vi "test1.vi"() -> ()   [LabVIEW 2019]
uses:
  <vilib>/measure/NI_MABase.lvlib
panel:
  in  "rate 2":dbl=500.0 format="%#_13g"
  in  "sampling info 6":cluster{"Fs":dbl, "#s":dbl}={"Fs"=2000.0, "#s"=100.0} {"Fs" format="%#_6f"; "#s" format="%#_6f"}
  in  "Back 3":T1={"Channel 1"={" frequency 1"=100, "signal type 1"=enum."Sine Wave", "amplitude 1"=1.5, "offset"=0.0, "phase"=0.0}, "Channel 2"={" frequency 1"=100, "signal type 1"=enum."Sine Wave", "amplitude 1"=1.5, "offset"=0.0, "phase"=90.0}, "Channel 3"={" frequency 1"=100, "signal type 1"=enum."Sine Wave", "amplitude 1"=1.5, "offset"=0, "phase"=180}, "Channel 4"={" frequency 1"=100, "signal type 1"=enum."Sine Wave", "amplitude 1"=1.5, "offset"=0.0, "phase"=270}}
  in  "rate":dbl=50.0 format="%#_13g"
  out "x-y":dbl=2.0449090003967285
  in  "sampling info 5":cluster{"Fs":dbl, "#s":dbl}={"Fs"=500000.0, "#s"=5000.0}
  in  "Back 2":T2={"Channel 1"={" frequency 1"=0, "signal type 1"=enum."Sine Wave", "amplitude 1"=0, "offset"=0.0, "phase"=0.0}, "Channel 2"={" frequency 1"=20000, "signal type 1"=enum."Sine Wave", "amplitude 1"=2.0, "offset"=0.0, "phase"=0.0}, "Channel 3"={" frequency 1"=20000, "signal type 1"=enum."Sine Wave", "amplitude 1"=2.0, "offset"=0, "phase"=0}, "Channel 4"={" frequency 1"=20000, "signal type 1"=enum."Sine Wave", "amplitude 1"=2.0, "offset"=0.0, "phase"=0}}
  in  "stop":bool
  out "Waveform Chart":waveform(dbl)[](graph)=[{"t0"=timestamp(0 s since 1904-01-01), "dt"=0.001, "Y"=[0.0, 1.8369701987210297e-16, -3.6739403974420594e-16, 5.51091059616309e-16, -7.347880794884119e-16, 9.18485099360515e-16, -1.102182119232618e-15, 1.285879139104721e-15, -1.469576158976824e-15, 1.653273178848927e-15, -1.83697019872103e-15, 2.020667218593133e-15, -2.204364238465236e-15, 2.388061258337339e-15, -2.5717582782094417e-15, 2.7554552980815448e-15, -2.9391523179536475e-15, 3.1228493378257506e-15, -3.3065463576978533e-15, 3.4902433775699565e-15, -3.673940397442059e-15, 3.857637417314163e-15, -4.0413344371862654e-15, 4.225031457058369e-15, -4.408728476930472e-15, 4.592425496802575e-15, -4.776122516674678e-15, 4.959819536546781e-15, -5.143516556418884e-15, 5.327213576290988e-15, -5.51091059616309e-15, 5.694607616035194e-15, -5.8783046359072966e-15, 6.0620016557794e-15, -6.245698675651503e-15, 6.429395695523606e-15, -6.613092715395709e-15, 6.7967897352678126e-15, -6.980486755139915e-15, 7.164183775012019e-15, -7.347880794884122e-15, 7.531577814756224e-15, -7.715274834628327e-15, 7.89897185450043e-15, -8.082668874372532e-15, 8.266365894244635e-15, -8.450062914116738e-15, 8.63375993398884e-15, -8.817456953860943e-15, 9.001153973733046e-15, -9.184850993605149e-15, 9.368548013477251e-15, -9.552245033349354e-15, 9.735942053221457e-15, -9.91963907309356e-15, 1.0103336092965662e-14, -1.0287033112837765e-14, 1.0470730132709868e-14, -1.065442715258197e-14, 1.0838124172454073e-14, -1.1021821192326176e-14, 1.1205518212198279e-14, -1.1389215232070381e-14, 1.1572912251942484e-14, -1.1756609271814587e-14, 1.194030629168669e-14, -1.2124003311558792e-14, 1.2307700331430895e-14, -1.2491397351302998e-14, 1.26750943711751e-14, -1.2858791391047203e-14, 1.3042488410919306e-14, -1.3226185430791409e-14, 1.3409882450663511e-14, -1.3593579470535614e-14, 1.3777276490407717e-14, -1.396097351027982e-14, 1.4144670530151922e-14, -1.4328367550024025e-14, 1.4512064569896128e-14, -1.469576158976823e-14, 1.4879458609640333e-14, -1.5063155629512436e-14, 1.524685264938454e-14, -1.543054966925664e-14, 1.5614246689128744e-14, -1.5797943709000847e-14, 1.598164072887295e-14, -1.6165337748745052e-14, 1.6349034768617155e-14, -1.6532731788489258e-14, 1.671642880836136e-14, -1.6900125828233463e-14, 1.7083822848105566e-14, -1.726751986797767e-14, 1.745121688784977e-14, -1.7634913907721874e-14, 1.7818610927593977e-14, -1.800230794746608e-14, 1.8186004967338182e-14]}, {"t0"=timestamp(0 s since 1904-01-01), "dt"=0.001, "Y"=[1.5, -1.5, 1.5, -1.5, 1.5, -1.5, 1.5, -1.5, 1.5, -1.5, 1.5, -1.5, 1.5, -1.5, 1.5, -1.5, 1.5, -1.5, 1.5, -1.5, 1.5, -1.5, 1.5, -1.5, 1.5, -1.5, 1.5, -1.5, 1.5, -1.5, 1.5, -1.5, 1.5, -1.5, 1.5, -1.5, 1.5, -1.5, 1.5, -1.5, 1.5, -1.5, 1.5, -1.5, 1.5, -1.5, 1.5, -1.5, 1.5, -1.5, 1.5, -1.5, 1.5, -1.5, 1.5, -1.5, 1.5, -1.5, 1.5, -1.5, 1.5, -1.5, 1.5, -1.5, 1.5, -1.5, 1.5, -1.5, 1.5, -1.5, 1.5, -1.5, 1.5, -1.5, 1.5, -1.5, 1.5, -1.5, 1.5, -1.5, 1.5, -1.5, 1.5, -1.5, 1.5, -1.5, 1.5, -1.5, 1.5, -1.5, 1.5, -1.5, 1.5, -1.5, 1.5, -1.5, 1.5, -1.5, 1.5, -1.5]}, {"t0"=timestamp(0 s since 1904-01-01), "dt"=0.001, "Y"=[1.8369701987210297e-16, -3.6739403974420594e-16, 5.51091059616309e-16, -7.347880794884119e-16, 9.18485099360515e-16, -1.102182119232618e-15, 1.285879139104721e-15, -1.469576158976824e-15, 1.653273178848927e-15, -1.83697019872103e-15, 2.020667218593133e-15, -2.204364238465236e-15, 2.388061258337339e-15, -2.5717582782094417e-15, 2.7554552980815448e-15, -2.9391523179536475e-15, 3.1228493378257506e-15, -3.3065463576978533e-15, 3.4902433775699565e-15, -3.673940397442059e-15, 3.857637417314163e-15, -4.0413344371862654e-15, 4.225031457058369e-15, -4.408728476930472e-15, 4.592425496802575e-15, -4.776122516674678e-15, 4.959819536546781e-15, -5.143516556418884e-15, 5.327213576290988e-15, -5.51091059616309e-15, 5.694607616035194e-15, -5.8783046359072966e-15, 6.0620016557794e-15, -6.245698675651503e-15, 6.429395695523606e-15, -6.613092715395709e-15, 6.7967897352678126e-15, -6.980486755139915e-15, 7.164183775012019e-15, -7.347880794884122e-15, 7.531577814756224e-15, -7.715274834628327e-15, 7.89897185450043e-15, -8.082668874372532e-15, 8.266365894244635e-15, -8.450062914116738e-15, 8.63375993398884e-15, -8.817456953860943e-15, 9.001153973733046e-15, -9.184850993605149e-15, 9.368548013477251e-15, -9.552245033349354e-15, 9.735942053221457e-15, -9.91963907309356e-15, 1.0103336092965662e-14, -1.0287033112837765e-14, 1.0470730132709868e-14, -1.065442715258197e-14, 1.0838124172454073e-14, -1.1021821192326176e-14, 1.1205518212198279e-14, -1.1389215232070381e-14, 1.1572912251942484e-14, -1.1756609271814587e-14, 1.194030629168669e-14, -1.2124003311558792e-14, 1.2307700331430895e-14, -1.2491397351302998e-14, 1.26750943711751e-14, -1.2858791391047203e-14, 1.3042488410919306e-14, -1.3226185430791409e-14, 1.3409882450663511e-14, -1.3593579470535614e-14, 1.3777276490407717e-14, -1.396097351027982e-14, 1.4144670530151922e-14, -1.4328367550024025e-14, 1.4512064569896128e-14, -1.469576158976823e-14, 1.4879458609640333e-14, -1.5063155629512436e-14, 1.524685264938454e-14, -1.543054966925664e-14, 1.5614246689128744e-14, -1.5797943709000847e-14, 1.598164072887295e-14, -1.6165337748745052e-14, 1.6349034768617155e-14, -1.6532731788489258e-14, 1.671642880836136e-14, -1.6900125828233463e-14, 1.7083822848105566e-14, -1.726751986797767e-14, 1.745121688784977e-14, -1.7634913907721874e-14, 1.7818610927593977e-14, -1.800230794746608e-14, 1.8186004967338182e-14, -1.8369701987210285e-14]}, {"t0"=timestamp(0 s since 1904-01-01), "dt"=0.001, "Y"=[-1.5, 1.5, -1.5, 1.5, -1.5, 1.5, -1.5, 1.5, -1.5, 1.5, -1.5, 1.5, -1.5, 1.5, -1.5, 1.5, -1.5, 1.5, -1.5, 1.5, -1.5, 1.5, -1.5, 1.5, -1.5, 1.5, -1.5, 1.5, -1.5, 1.5, -1.5, 1.5, -1.5, 1.5, -1.5, 1.5, -1.5, 1.5, -1.5, 1.5, -1.5, 1.5, -1.5, 1.5, -1.5, 1.5, -1.5, 1.5, -1.5, 1.5, -1.5, 1.5, -1.5, 1.5, -1.5, 1.5, -1.5, 1.5, -1.5, 1.5, -1.5, 1.5, -1.5, 1.5, -1.5, 1.5, -1.5, 1.5, -1.5, 1.5, -1.5, 1.5, -1.5, 1.5, -1.5, 1.5, -1.5, 1.5, -1.5, 1.5, -1.5, 1.5, -1.5, 1.5, -1.5, 1.5, -1.5, 1.5, -1.5, 1.5, -1.5, 1.5, -1.5, 1.5, -1.5, 1.5, -1.5, 1.5, -1.5, 1.5]}]
  in  "Back":T1={"Channel 1"={" frequency 1"=500, "signal type 1"=enum."Sine Wave", "amplitude 1"=1.5, "offset"=0.0, "phase"=0.0}, "Channel 2"={" frequency 1"=500, "signal type 1"=enum."Sine Wave", "amplitude 1"=1.5, "offset"=0.0, "phase"=90.0}, "Channel 3"={" frequency 1"=500, "signal type 1"=enum."Sine Wave", "amplitude 1"=1.5, "offset"=0, "phase"=180}, "Channel 4"={" frequency 1"=500, "signal type 1"=enum."Sine Wave", "amplitude 1"=1.5, "offset"=0.0, "phase"=270}}
  in  "sampling info 4":cluster{"Fs":dbl, "#s":dbl}={"Fs"=1000.0, "#s"=100.0} {"Fs" format="%#_6f"; "#s" format="%#_6f"}
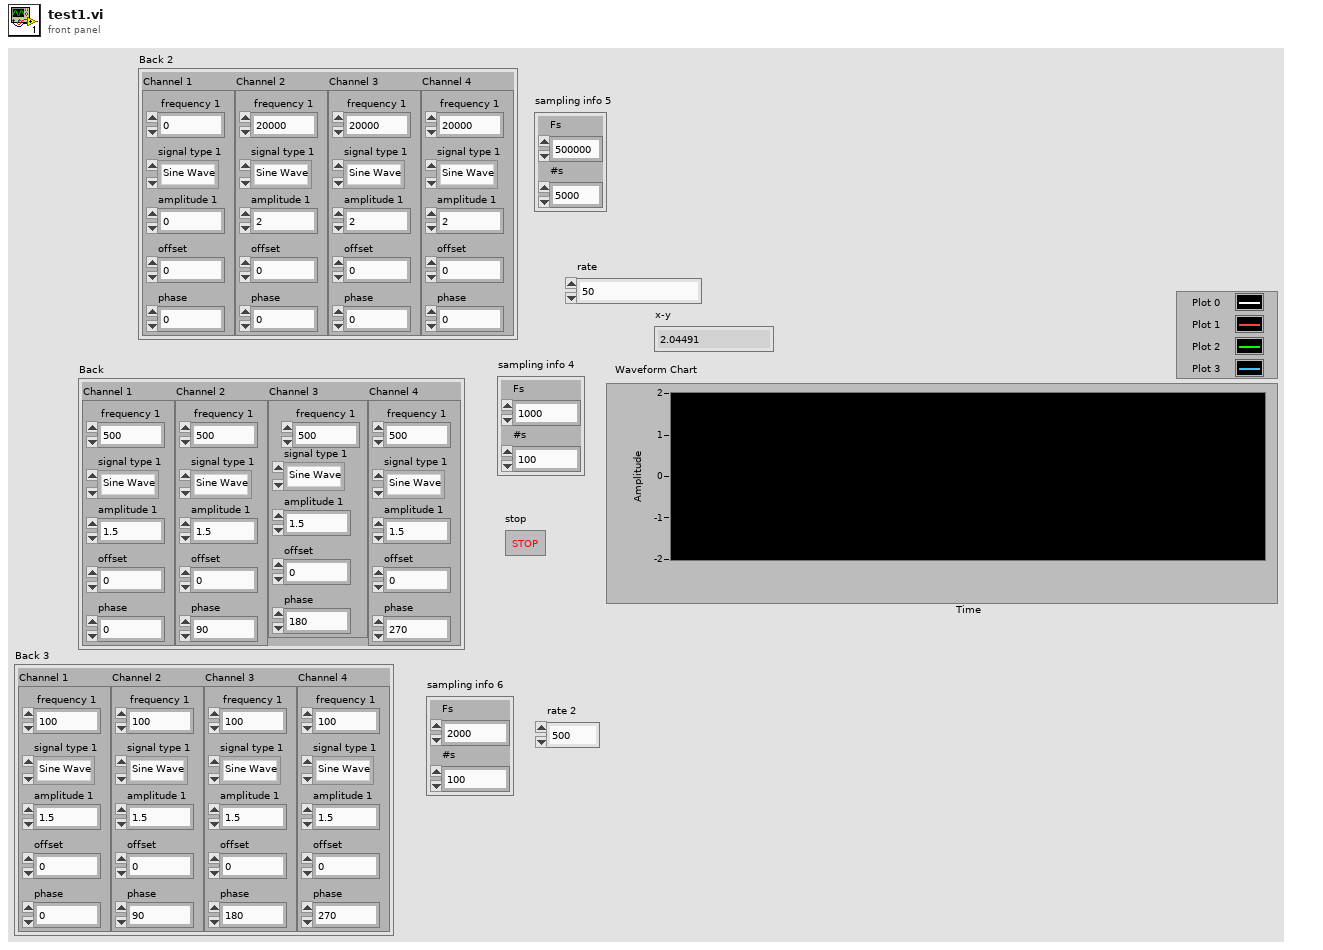
[diagram p1: front panel]
types:
  T1 = cluster{"Channel 1":cluster{" frequency 1":i32, "signal type 1":enum16{"Sine Wave", "Triangle Wave", "Square Wave", "Sawtooth Wave"}, "amplitude 1":dbl, "offset":dbl, "phase":dbl}, "Channel 2":cluster{" frequency 1":i32, "signal type 1":enum16{"Sine Wave", "Triangle Wave", "Square Wave", "Sawtooth Wave"}, "amplitude 1":dbl, "offset":dbl, "phase":dbl}, "Channel 3":cluster{" frequency 1":i32, "signal type 1":enum16{"Sine Wave", "Triangle Wave", "Square Wave", "Sawtooth Wave"}, "amplitude 1":dbl, "offset":i32, "phase":i32}, "Channel 4":cluster{" frequency 1":i32, "signal type 1":enum16{"Sine Wave", "Triangle Wave", "Square Wave", "Sawtooth Wave"}, "amplitude 1":dbl, "offset":dbl, "phase":i32}}
  T2 = cluster{"Channel 1":cluster{" frequency 1":i32, "signal type 1":enum16{"Sine Wave", "Triangle Wave", "Square Wave", "Sawtooth Wave"}, "amplitude 1":i32, "offset":dbl, "phase":dbl}, "Channel 2":cluster{" frequency 1":i32, "signal type 1":enum16{"Sine Wave", "Triangle Wave", "Square Wave", "Sawtooth Wave"}, "amplitude 1":dbl, "offset":dbl, "phase":dbl}, "Channel 3":cluster{" frequency 1":i32, "signal type 1":enum16{"Sine Wave", "Triangle Wave", "Square Wave", "Sawtooth Wave"}, "amplitude 1":dbl, "offset":i32, "phase":i32}, "Channel 4":cluster{" frequency 1":i32, "signal type 1":enum16{"Sine Wave", "Triangle Wave", "Square Wave", "Sawtooth Wave"}, "amplitude 1":dbl, "offset":dbl, "phase":i32}}
  T3 = cluster{" frequency 1":i32, "signal type 1":enum16{"Sine Wave", "Triangle Wave", "Square Wave", "Sawtooth Wave"}, "amplitude 1":dbl, "offset":dbl, "phase":dbl}
  T4 = cluster{" frequency 1":i32, "signal type 1":enum16{"Sine Wave", "Triangle Wave", "Square Wave", "Sawtooth Wave"}, "amplitude 1":dbl, "offset":i32, "phase":i32}
  T5 = cluster{" frequency 1":i32, "signal type 1":enum16{"Sine Wave", "Triangle Wave", "Square Wave", "Sawtooth Wave"}, "amplitude 1":dbl, "offset":dbl, "phase":i32}
  T6 = cluster{" frequency 1":i32, "signal type 1":enum16{"Sine Wave", "Triangle Wave", "Square Wave", "Sawtooth Wave"}, "amplitude 1":dbl, "offset":dbl, "phase":dbl}[]
  T7 = enum16{"Sine Wave", "Triangle Wave", "Square Wave", "Sawtooth Wave"}
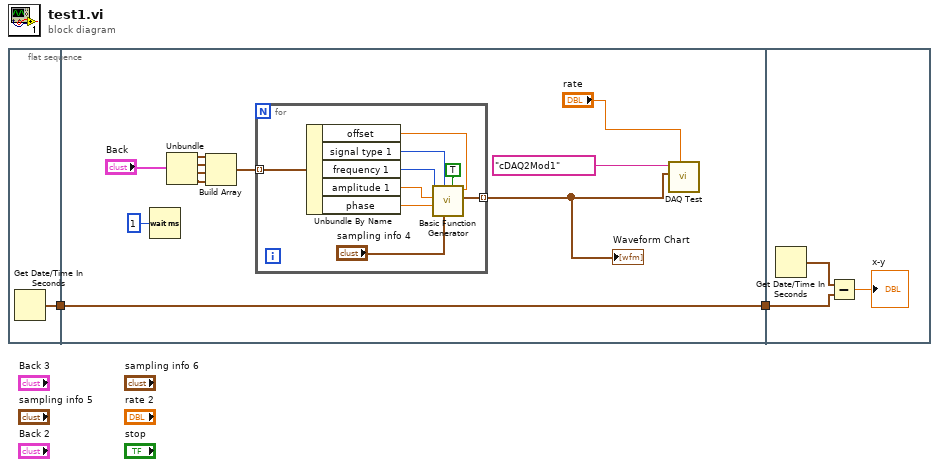
[diagram p0: block diagram]
diagram:
  n1 = flat-sequence {
    tunnel: [w3] -> w2
    tunnel: w2 -> [w7]
    tunnel: [w7] -> w1
    tunnel: w1 -> [w26]
    frame #0 {
      n2 = Get Date/Time In Seconds() -> (seconds since 1Jan1904=w3:timestamp)
    }
    frame #1 {
      n3 = Wait (ms)(milliseconds to wait=u32 1) -> ()  [unwired: 1 out]
      n4 = Unbundle("Back") -> ("Channel 1"=w10:T3, "Channel 2"=w11:T3, "Channel 3"=w12:T4, "Channel 4"=w13:T5)
      n5 = Build Array(w10, w11, w12, w13) -> (w9:T6)
      n6 = for {
        tunnel: w9 -> [w15] mode=indexing
        tunnel: [w16] -> w6 mode=indexing
        n7 = Unbundle By Name(w15) -> ("offset"=w17:dbl, "signal type 1"=w18:T7, "frequency 1"=w19:i32, "amplitude 1"=w20:dbl, "phase"=w21:dbl)
        n8 = call <vilib>:"Basic Function Generator.vi"("offset"=w17, "reset signal"=TRUE, "sampling info"="sampling info 4", "signal type"=w18, "phase"=w21, "amplitude"=w20, "frequency"=w19) -> ("signal out"=w16:waveform(dbl))  [unwired: 2 in, 2 out]
      }
      "Waveform Chart" <- w6
      n9 = call "DAQ Test.vi"("rate"="rate", "data"=w6, "device name"=tag "cDAQ2Mod1") -> ()  [unwired: 7 in, 2 out]
    }
    frame #2 {
      n10 = Get Date/Time In Seconds() -> (seconds since 1Jan1904=w25:timestamp)
      n11 = Subtract(x=w25, y=w26) -> (x-y=→"x-y":dbl)
    }
  }
